vi "Controls.vi"() -> ()   [LabVIEW 2019]
panel:
  in  "String":string
  in  "Boolean":bool
  in  "Set Temp":dbl(slide) scale=0.0..100.0
  in  "Numeric":dbl
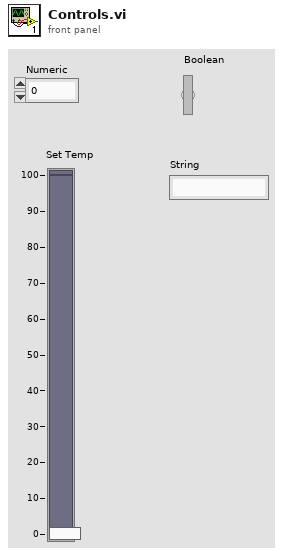
[diagram p1: front panel]
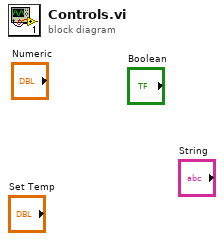
[diagram p0: block diagram]
diagram:
